vi "RANGE Check For Totalizer.vi"(7 "Calculated Totalizer":dbl, 10 "Meter Totalizer":dbl) -> (3 "Tot. Flow (Liters) out":dbl)   [LabVIEW 2023]
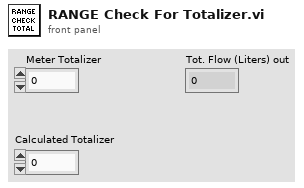
[diagram p1: front panel]
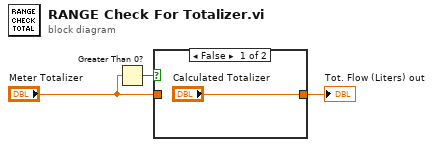
[diagram p0: block diagram]
diagram:
  n1 = Greater Than 0?(x="Meter Totalizer") -> (x > 0?=w1:bool)
  n2 = case shown="False" w1 {
    tunnel: ["Calculated Totalizer" w5] -> w3
    tunnel: "Meter Totalizer" -> [_ w5]
    frame False {
    }
    frame True {
    }
  }
  "Tot. Flow (Liters) out" <- w3
